vi "LoggingData.vi"(8 "error in (no error)":errorcluster, 10 "Start time":u32, 11 "Refmum":refnum<file>) -> (0 "error out":errorcluster, 3 "Byte Stream File out":refnum<file>)   [LabVIEW 2017]
uses:
  Framework/Robot Global Data.vi
  Drive/Implementation/Drive Published Globals.vi
  Elevator/Implementation/Elevator Published Globals.vi
  Intake/Implementation/Intake Published Globals.vi
  <vilib>/NI_Real-Time Target Support.lvlib
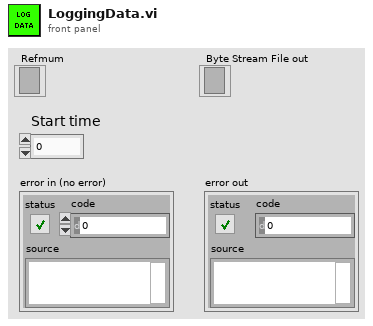
[diagram p1: front panel]
types:
  T1 = typedef "Z900_navX_Flags_OpStatusTypeDef.ctl" = u8
  T2 = typedef "Z900_navX_Flags_CalibrationStatusTypeDef.ctl" = u8
  T3 = cluster{"Update Rate Hz":u8, "Accelerometer Full-Scale Range":u8, "Gyro Full-Scale Range":u16, "OP Status":T1, "Calibration Status":T2, "Sensor Status":cluster{"MOVING":bool, "YAW_STABLE":bool, "MAG_DISTURBANCE":bool, "ALTITUDE_VALID":bool, "SEALEVEL_PRESS_SET":bool, "FUSED_HEADING_VALID":bool}, "Self Test Status":cluster{"Gyro Passed":bool, "Accel Passed":bool, "Mag Passed":bool, "Baro Passed":bool, "Complete":bool}}
  T4 = cluster{"MOVING":bool, "YAW_STABLE":bool, "MAG_DISTURBANCE":bool, "ALTITUDE_VALID":bool, "SEALEVEL_PRESS_SET":bool, "FUSED_HEADING_VALID":bool}
  T5 = cluster{"Yaw":dbl, "Roll":dbl, "Pitch":dbl, "Heading":dbl, "Fused Heading":dbl}
  T6 = typedef "WPI_DriverStationRobotMode2.ctl" = enum16{"Autonomous Disabled", "Autonomous Enabled", "Teleop Disabled", "Teleop Enabled", "Disconnected", "Finish", "Test Disabled", "Test Enabled", "Emergency Stopped"}
  T7 = typedef "NI_Real-Time Target Support.lvlib/RT CPU Load.ctl" = cluster{"Total (%)":dbl, "Time Critical (%)":dbl, "Timed Structures (%)":dbl, "High (%)":dbl, "Above Normal (%)":dbl, "Normal (%)":dbl, "Background (%)":dbl, "Idle (%)":dbl, "ISR (%)":dbl}
  T8 = cluster{"LinearAcceleration X":dbl, "LinearAcceleration Y":dbl, "LinearAcceleration Z":dbl}
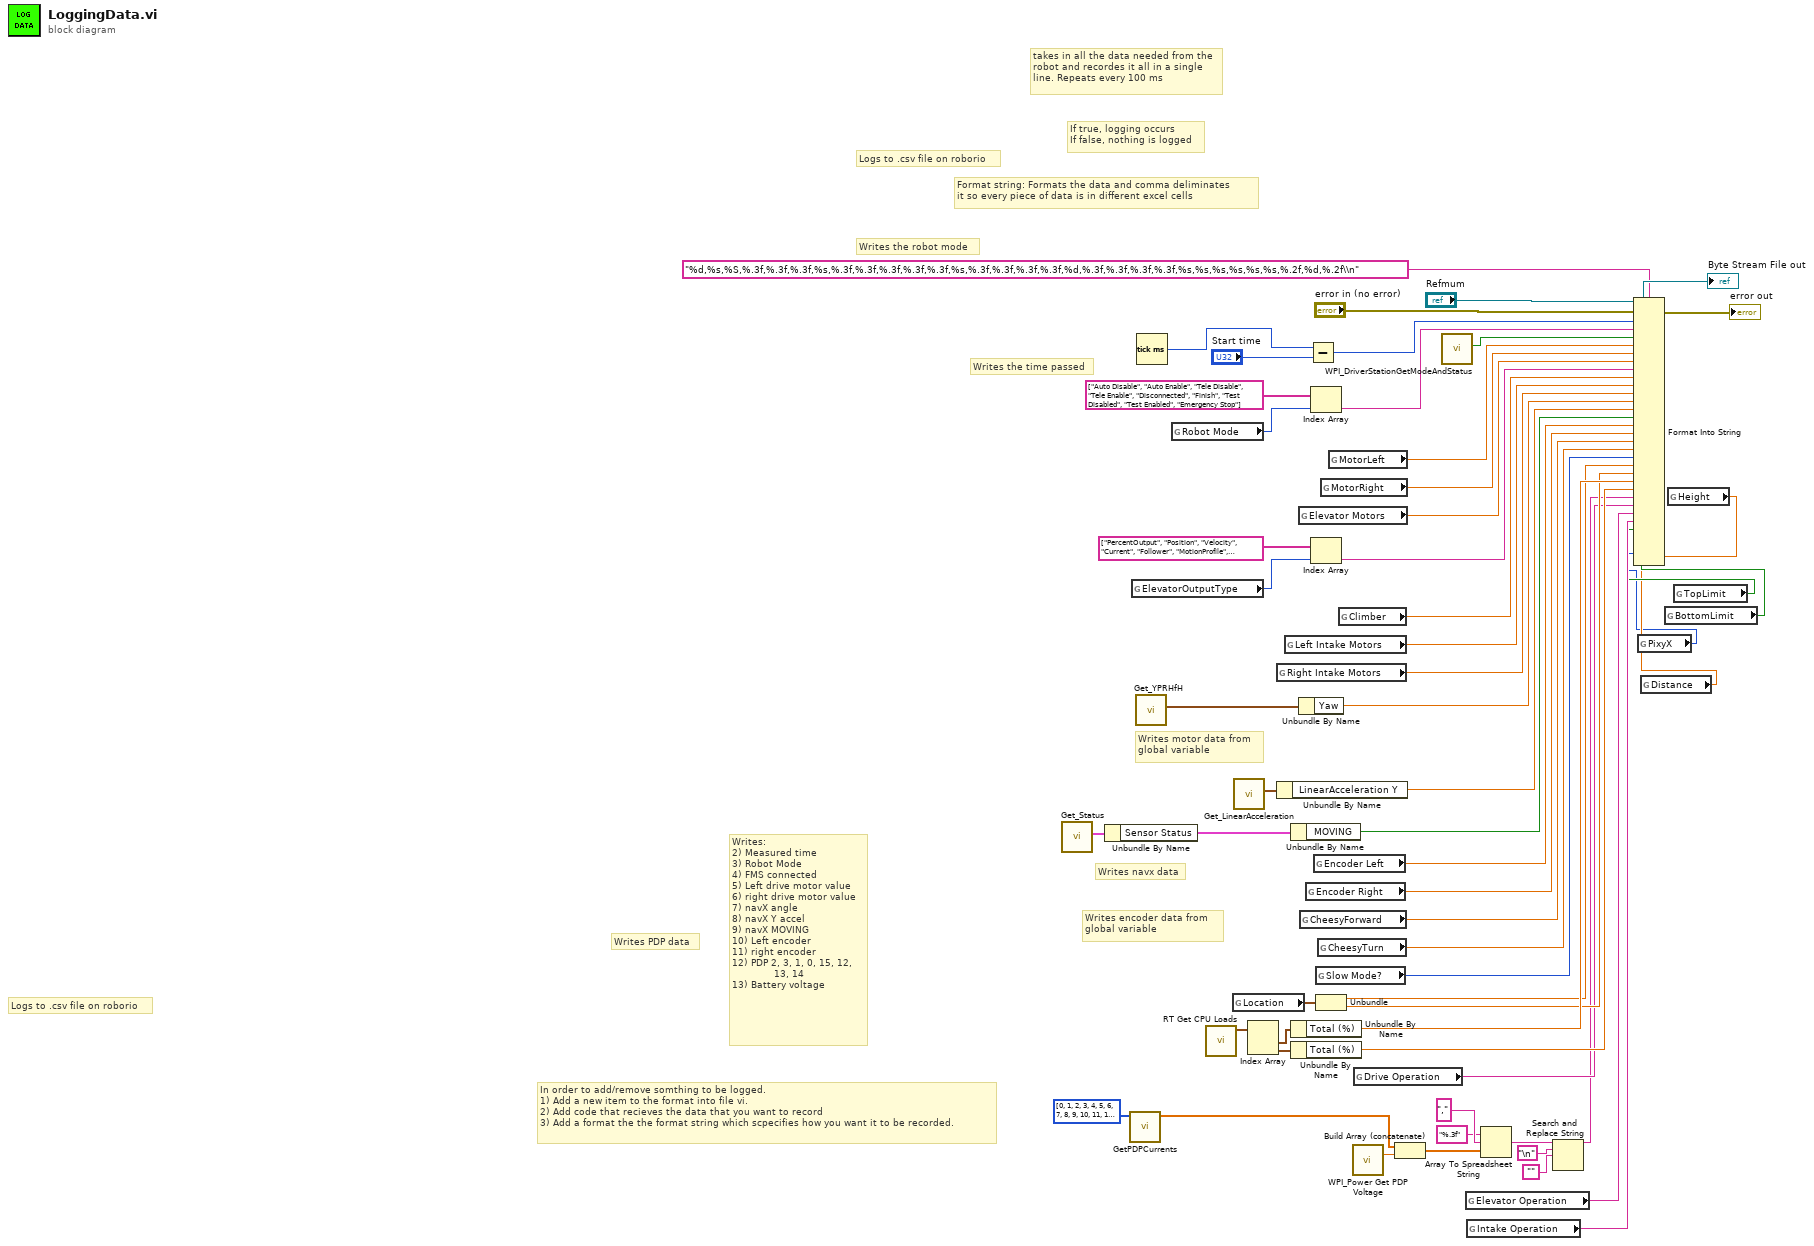
[diagram p0: block diagram]
diagram:
  # "Writes the time passed"
  # "Writes encoder data from \nglobal variable"
  # "Writes PDP data"
  # "Writes navx data"
  # "Writes motor data from\nglobal variable"
  # "Writes the robot mode"
  # "Logs to .csv file on roborio"
  # "Format string: Formats the data and comma deliminates \nit so every piece of data is in different excel cells"
  # "In order to add/remove somthing to be logged.\n1) Add a new item to the format into file vi.\n2) Add code that recieves the data that you want to record\n3) Add a format the the format string which scpecifies how you want it to be recorded."
  # "Logs to .csv file on roborio"
  # "If true, logging occurs\nIf false, nothing is logged"
  # "Writes:\n2) Measured time\n3) Robot Mode\n4) FMS connected\n5) Left drive motor value\n6) right drive motor value\n7) navX angle\n8) navX Y accel\n9) navX MOVING\n10) Left encoder\n11) right encoder\n12) PDP 2, 3, 1, 0, 15, 12,\n              13, 14\n13) Battery voltage"
  # "takes in all the data needed from the robot and recordes it all in a single line. Repeats every 100 ms"
  n1 = call <vilib>:"Get_Status.vi"() -> ("Status"=w46:T3)  [unwired: 11 in]
  n2 = Unbundle By Name(w46) -> ("Sensor Status"=w47:T4)
  n3 = call "GetPDPCurrents.vi"("Channels"=i32[] [0, 1, 2, 3, 4, 5, 6, 7, 8, 9, 10, 11, 12, 13, 14, 15]) -> ("Currents"=w55:dbl[])  [unwired: 10 in]
  n4 = global read "Robot Global Data.vi" "ElevatorOutputType"() -> (w31:enum16{""})
  n5 = call <vilib>:"Get_YPRHfH.vi"() -> ("YRPHfH"=w37:T5)  [unwired: 11 in]
  n6 = Tick Count (ms)() -> (millisecond timer value=w39:u32)
  n7 = global read "Robot Global Data.vi" "Robot Mode"() -> (w43:T6)
  n8 = call <vilib>:"RT Get CPU Loads.vi"() -> ("CPU loads"=w48:T7[])  [unwired: 10 in, 1 out]
  n9 = global read "Drive Published Globals.vi" "Location"() -> (w42:cluster{dbl, dbl})
  n10 = call <vilib>:"Get_LinearAcceleration.vi"() -> ("Linear Acceleration"=w41:T8)  [unwired: 11 in]
  n11 = Index Array(array=w48) -> (element #1=w50:T7, element #2=w49:T7)  [unwired: 2 in]
  n12 = global read "Robot Global Data.vi" "Right Intake Motors"() -> (w16:dbl)
  n13 = Unbundle By Name(w41) -> ("LinearAcceleration Y"=w19:dbl)
  n14 = global read "Robot Global Data.vi" "Left Intake Motors"() -> (w15:dbl)
  n15 = Unbundle By Name(w47) -> ("MOVING"=w18:bool)
  n16 = Unbundle By Name(w50) -> ("Total (%)"=w27:dbl)
  n17 = Unbundle By Name(w49) -> ("Total (%)"=w28:dbl)
  n18 = global read "Robot Global Data.vi" "Elevator Motors"() -> (w30:dbl)
  n19 = Unbundle By Name(w37) -> ("Yaw"=w17:dbl)
  n20 = global read "Robot Global Data.vi" "CheesyForward"() -> (w22:dbl)
  n21 = global read "Drive Published Globals.vi" "Encoder Right"() -> (w21:dbl)
  n22 = Subtract(x=w39, y="Start time") -> (x-y=w40:u32)
  n23 = Index Array(array=string[] ["Auto Disable", "Auto Enable", "Tele Disable", "Tele Enable", "Disconnected", "Finish", "Test Disabled", "Test Enabled", "Emergency Stop"], index=w43) -> (element=w45:string)
  n24 = Index Array(array=string[] ["PercentOutput", "Position", "Velocity", "Current", "Follower", "MotionProfile", "MotionMagic", "MotionMagicArc", "MotionProfileArc", "Disabled"] ("Strings []"), index=w31) -> (element=w29:string)
  n25 = global read "Drive Published Globals.vi" "Encoder Left"() -> (w20:dbl)
  n26 = global read "Robot Global Data.vi" "Slow Mode?"() -> (w24:u32)
  n27 = Unbundle(w42) -> (w25:dbl, w26:dbl)
  n28 = global read "Robot Global Data.vi" "CheesyTurn"() -> (w23:dbl)
  n29 = global read "Drive Published Globals.vi" "MotorRight"() -> (w32:dbl)
  n30 = global read "Drive Published Globals.vi" "MotorLeft"() -> (w34:dbl)
  n31 = global read "Robot Global Data.vi" "Climber"() -> (w14:dbl)
  n32 = call <vilib>:"WPI_Power Get PDP Voltage.vi"() -> ("voltage (V)"=w53:dbl)  [unwired: 14 in, 1 out]
  n33 = global read "Robot Global Data.vi" "Drive Operation"() -> (w11:string)
  n34 = Build Array (concatenate)(w55, w53) -> (w56:dbl[])
  n35 = call <vilib>:"WPI_DriverStationGetModeAndStatus.vi"() -> ("FMS Attached"=w36:bool)  [unwired: 10 in, 1 out]
  n36 = global read "Robot Global Data.vi" "Elevator Operation"() -> (w12:string)
  n37 = global read "Robot Global Data.vi" "Intake Operation"() -> (w13:string)
  n38 = Array To Spreadsheet String(delimiter (Tab)=",", array=w56, 3:"%.3f" ("format string")) -> (spreadsheet string=w8:string)
  n39 = Search and Replace String(input string=w8, search string="\n", replace string="") -> (result string=w6:string)  [unwired: 5 in, 3 out]
  n40 = global read "Drive Published Globals.vi" "PixyX"() -> (w1:i32)
  n41 = global read "Intake Published Globals.vi" "Distance"() -> (w2:dbl)
  n42 = global read "Elevator Published Globals.vi" "BottomLimit"() -> (w4:bool)
  n43 = global read "Elevator Published Globals.vi" "Height"() -> (w3:dbl)
  n44 = global read "Elevator Published Globals.vi" "TopLimit"() -> (w5:bool)
  n45 = Format Into String(format string="%d,%s,%S,%.3f,%.3f,%.3f,%s,%.3f,%.3f,%.3f,%.3f,%.3f,%s,%.3f,%.3f,%.3f,%.3f,%d,%.3f,%.3f,%.3f,%.3f,%s,%s,%s,%s,%s,%s,%.2f,%d,%.2f\\n", initial string="Refmum", error in="error in (no error)", w40, w45, w36, w34, w32, w30, w29, w14, w15, w16, w17, w19, w18, w20, w21, w22, w23, w24, w25, w26, w27, w28, w6, w11, w12, w13, w5, w4, w3, w1, w2) -> (resulting string=→"Byte Stream File out":refnum<file>, error out=→"error out":errorcluster)
